vi "Analyse.vi"(8 "error in (no error)":errorcluster, 10 "ImageData":T1, 11 "FluorescenceLiveAnalyser in":refnum<class "FluorescenceLiveAnalyser.lvclass">) -> (0 "error out":errorcluster, 3 "FluorescenceLiveAnalyser out":refnum<class "FluorescenceLiveAnalyser.lvclass">)   [LabVIEW 2011, in "Tools.lvlib" / "Imaging.lvlib" / "FluorescenceLiveAnalyser.lvclass"]
uses:
  FluorescenceLiveAnalyser.lvclass
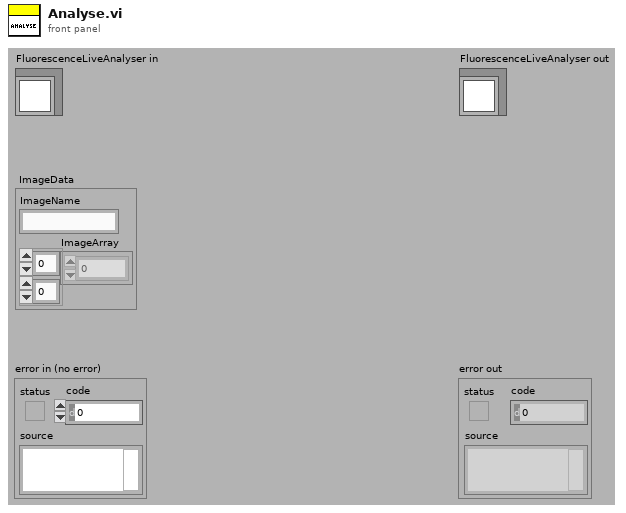
[diagram p1: front panel]
types:
  T1 = cluster{"ImageName":string, "ImageArray":sgl[][]}
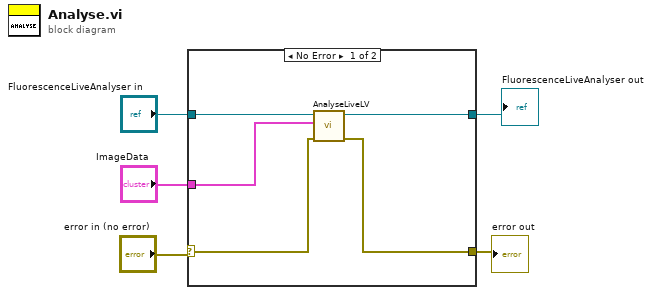
[diagram p0: block diagram]
diagram:
  n1 = case shown="No Error" "error in (no error)" {
    selector: "error in (no error)" -> [w7 w11]
    tunnel: "FluorescenceLiveAnalyser in" -> [w10 w12]
    tunnel: [w9 w12] -> w3
    tunnel: [w6 w11] -> w2
    tunnel: "ImageData" -> [w8 _]
    frame No Error {
      n2 = call "AnalyseLiveLV.vi"("error in (no error)"=w7, "ImageData"=w8, "FluorescenceLiveAnalyser in"=w10) -> ("error out"=w6:errorcluster, "FluorescenceLiveAnalyser out"=w9:refnum<class "FluorescenceLiveAnalyser.lvclass">)  [unwired: 7 in]
    }
    frame Error {
    }
  }
  "error out" <- w2
  "FluorescenceLiveAnalyser out" <- w3
